vi "Set TCP Settings.vi"(7 "Timeout":i32, 8 "error in (no error)":errorcluster, 9 "Port":u16, 10 "Address":string, 11 "Item Ref in":T1 format="%.0x") -> (0 "error out":errorcluster, 3 "Item Ref out":T1 format="%.0x")   [LabVIEW 2021, in "Modbus Master System Explorer.lvlib"]
uses:
  Modbus Master System Explorer.lvlib
  <vilib>/NI VeriStand/Custom Device API/Custom Device Item Ref.ctl
  Shared/Constants.vi
  <vilib>/NI VeriStand/Custom Device API/Set Item Property (String).vi
  <vilib>/NI VeriStand/Custom Device API/Set Item Property (U16).vi
  <vilib>/NI VeriStand/Custom Device API/Set Item Property (I32).vi
  <vilib>/NI VeriStand/Custom Device API/Custom Device API.lvlib
  Shared/Modbus Master Shared.lvlib
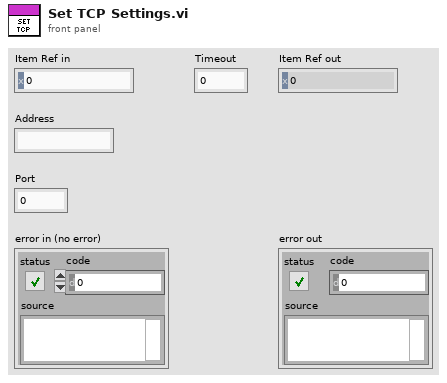
[diagram p1: front panel]
types:
  T1 = typedef "Custom Device API.lvlib/Custom Device Item Ref.ctl" = u64
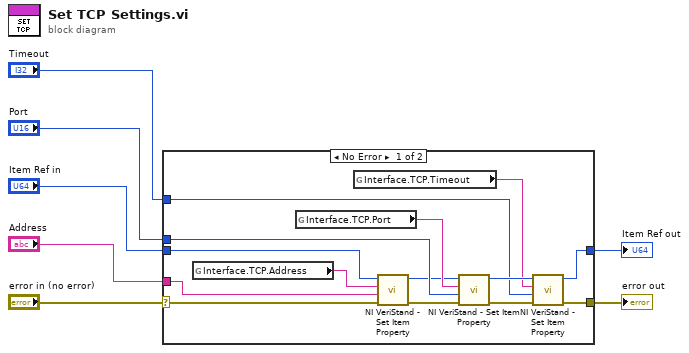
[diagram p0: block diagram]
diagram:
  n1 = case shown="No Error" "error in (no error)" {
    selector: "error in (no error)" -> [w14 w23]
    tunnel: [w11 w23] -> w7
    tunnel: [w10 w22] -> w6
    tunnel: "Port" -> [w21 _]
    tunnel: "Address" -> [w17 _]
    tunnel: "Item Ref in" -> [w15 w22]
    tunnel: "Timeout" -> [w8 _]
    frame No Error {
      n2 = global read "Constants.vi" "Interface.TCP.Address"() -> (w16:string)
      n3 = global read "Constants.vi" "Interface.TCP.Port"() -> (w20:string)
      n4 = global read "Constants.vi" "Interface.TCP.Timeout"() -> (w9:string)
      n5 = call-poly <vilib>:"NI VeriStand - Set Item Property.vi"("error in (no error)"=w14, "Value"=w17, "Property Name"=w16, "Item Ref in"=w15) -> ("error out"=w18:errorcluster, "Item Ref out"=w19:T1)  [unwired: 5 in, 1 out]
      n6 = call-poly <vilib>:"NI VeriStand - Set Item Property.vi"("error in (no error)"=w18, "Value"=w21, "Property Name"=w20, "Item Ref in"=w19) -> ("error out"=w13:errorcluster, "Item Ref out"=w12:T1)  [unwired: 5 in, 1 out]
      n7 = call-poly <vilib>:"NI VeriStand - Set Item Property.vi"("error in (no error)"=w13, "Value"=w8, "Property Name"=w9, "Item Ref in"=w12) -> ("error out"=w11:errorcluster, "Item Ref out"=w10:T1)  [unwired: 5 in, 1 out]
    }
    frame Error {
    }
  }
  "error out" <- w7
  "Item Ref out" <- w6
